vi "ConstantSignalMessage.vi"(6 "Filter":T1=enum."NoFilter", 7 "OutputStage":T2, 9 "Offset":dbl, 10 "DC Value":dbl, 11 "Duration":dbl) -> (3 "ConstantSignalMessage":string)   [LabVIEW 2019]
uses:
  OutputStageTypeDef.ctl
  FilterTypeDef.ctl
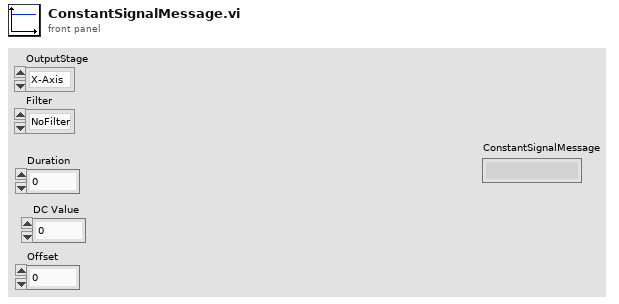
[diagram p1: front panel]
types:
  T1 = typedef "FilterTypeDef.ctl" = enum16{"IIR_X", "IIR_Y", "NoFilter", "Bessel6thOrder300"}
  T2 = typedef "OutputStageTypeDef.ctl" = enum16{"X-Axis", "Y-Axis"}
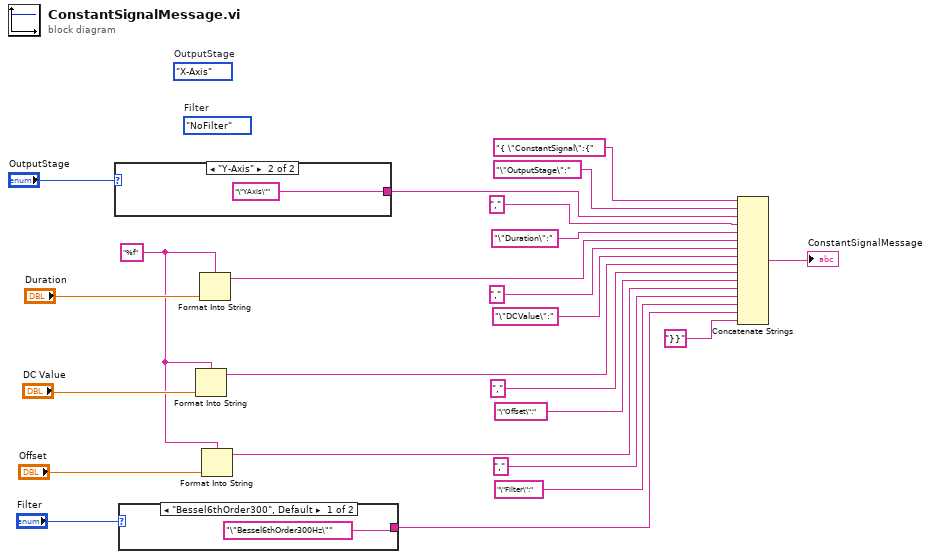
[diagram p0: block diagram]
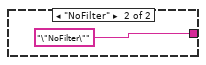
[diagram p2: hidden frame]
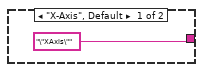
[diagram p3: hidden frame]
diagram:
  w1 = "%f" ("format string")
  (unwired) OutputStageTypeDef."X-Axis"  # OutputStage
  (unwired) FilterTypeDef."NoFilter"  # Filter
  n1 = case shown="\"Y-Axis\"" "OutputStage" {
    tunnel: ["\"XAxis\"" "\"YAxis\""] -> w15
    frame "X-Axis", Default {
    }
    frame "Y-Axis" {
    }
  }
  n2 = case shown="\"Bessel6thOrder300\", Default" "Filter" {
    tunnel: ["\"Bessel6thOrder300Hz\"" "\"NoFilter\""] -> w3
    frame "Bessel6thOrder300", Default {
    }
    frame "NoFilter" {
    }
  }
  n3 = Format Into String(format string=w1, "DC Value") -> (resulting string=w9:string)  [unwired: 2 in, 1 out]
  n4 = Format Into String(format string=w1, "Duration") -> (resulting string=w12:string)  [unwired: 2 in, 1 out]
  n5 = Format Into String(format string=w1, "Offset") -> (resulting string=w6:string)  [unwired: 2 in, 1 out]
  n6 = Concatenate Strings("{ \"ConstantSignal\":{", "\"OutputStage\":", w15, ",", "\"Duration\":", w12, ",", "\"DCValue\":", w9, ",", "\"Offset\":", w6, ",", "\"Filter\":", w3, "}}" ("string")) -> (→"ConstantSignalMessage":string)
